vi "initialize_data_log.vi"(7 "Overwrite?":bool, 8 "error in (no error)":errorcluster, 9 "Initialization Data":variant, 10 "Path":path, 11 "pcfs_hdf5_log in":refnum<class "pcfs_hdf5_log.lvclass">) -> (0 "error out":errorcluster, 3 "pcfs_hdf5_log out":refnum<class "pcfs_hdf5_log.lvclass">)   [LabVIEW 2015, in "pcfs_hdf5_log.lvclass"]
uses:
  pcfs_hdf5_log.lvclass
  Detector_Class/Picoquant/Hydraharp/hydraharp_panel/hpanel_acq_modes.ctl
  pcfs_hdf5_log.lvclass/pcfs_hdf5_log.ctl
  <vilib>/UPVI/lvhdf5/file.llb/LVH5F Operation.ctl
  Detector_Class/Picoquant/Hydraharp/hydraharp/hydraharp.lvclass
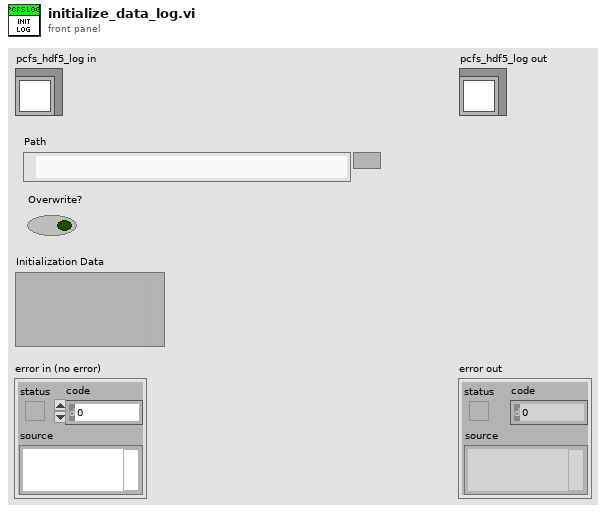
[diagram p1: front panel]
types:
  T1 = typedef "hpanel_acq_modes.ctl" = u16
  T2 = typedef "LVH5F Operation.ctl" = enum16{"open", "open or create", "create or replace", "create or replace (with confirmation)", "create", "open (read only)"}
  T3 = typedef "HDF5 Ref.ctl" = refnum<k1>
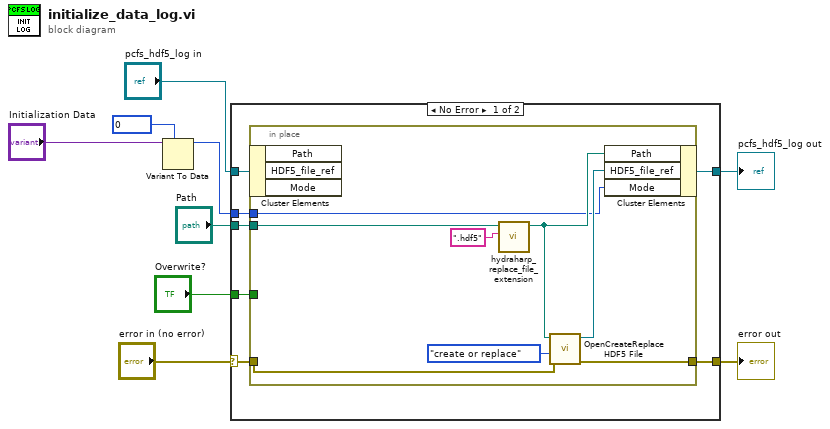
[diagram p0: block diagram]
diagram:
  w2 = T1 0 items=["T2"=2, "T3"=3] ("Mode")
  n1 = Variant To Data(type=w2, Variant="Initialization Data") -> (data=w1:T1)  [unwired: 1 in, 1 out]
  n2 = case shown="No Error" "error in (no error)" {
    selector: "error in (no error)" -> [w15 w26]
    tunnel: "pcfs_hdf5_log in" -> [w16 w25]
    tunnel: "Path" -> [w14 _]
    tunnel: "Overwrite?" -> [w13 _]
    tunnel: [w12 w25] -> w5
    tunnel: [w11 w26] -> w4
    tunnel: w1 -> [w10 _]
    frame No Error {
      n3 = in-place {
        in-place-border: w15 -> [w24]
        in-place-border: w14 -> [w23]
        in-place-border: w13 -> [_]
        in-place-border: [w19] -> w11
        in-place-border: w10 -> [w18]
        n4 = in-place-cluster #1(w16) -> ()  [unwired: 3 out]
        n5 = call "hydraharp_replace_file_extension.vi"("new_extension"=".hdf5", "input_file"=w23) -> ("new_name"=w20:path)  [unwired: 9 in]
        n6 = call <vilib>:"OpenCreateReplace HDF5 File.vi"("error in (no error)"=w24, "function (open or create)"=LVH5F_Operation."create or replace", "path"=w20) -> ("error out"=w19:errorcluster, "HDF5 Ref out"=w21:T3)  [unwired: 5 in]
        n7 = in-place-cluster #1("Path"=w20, "HDF5_file_ref"=w21, "Mode"=w18) -> (w12:refnum<class "pcfs_hdf5_log.lvclass">)
      }
    }
    frame Error {
    }
  }
  "error out" <- w4
  "pcfs_hdf5_log out" <- w5
